vi "Cannon Angle Set.vi"(11 "Angle Set Point":dbl(knob) scale=0.0..200.0) -> (2 "On Target":bool, 3 "zAvit Vbus Out":dbl)   [LabVIEW 2012]
uses:
  BotStatus.vi
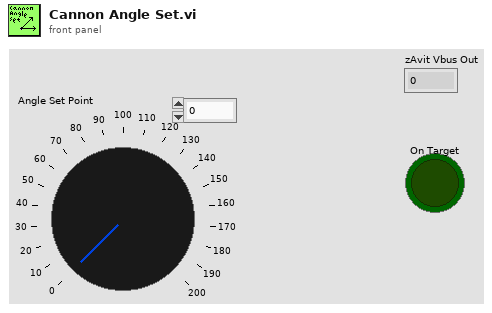
[diagram p1: front panel]
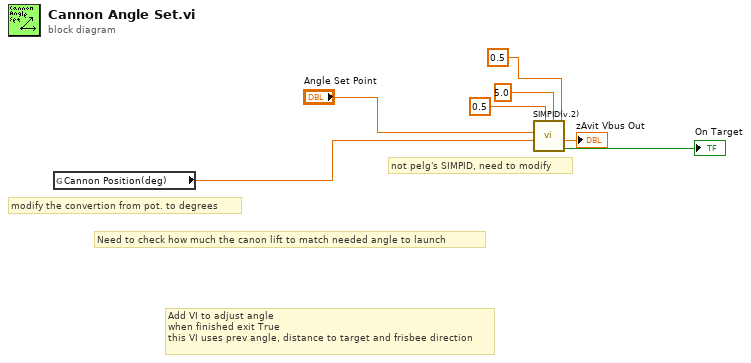
[diagram p0: block diagram]
diagram:
  # "not pelg's SIMPID, need to modify"
  # "Need to check how much the canon lift to match needed angle to launch"
  # "modify the convertion from pot. to degrees"
  # "Add VI to adjust angle\nwhen finished exit True\nthis VI uses prev angle, distance to target and frisbee direction"
  n1 = global read "BotStatus.vi" "Cannon Position(deg)"() -> (w4:dbl)
  n2 = call "SIMPID(v.2).vi"("Range"=0.5, "upper limit"=5.0, "lower limit"=0.5, "Current Point"=w4, "Set Point"="Angle Set Point") -> ("On Target"=→"On Target":bool, "result"=→"zAvit Vbus Out":dbl)  [unwired: 5 in]
